vi "reconstruction_error.vi"(8 "error in (no error)":errorcluster caption="entrée d'erreur (pas d'erreur)", 11 "Isomap.lvclass":refnum<class "Isomap.lvclass">) -> (0 "error out":errorcluster caption="sortie d'erreur", 2 "reconstruction_error":dbl, 3 "Isomap.lvclass 2":refnum<class "Isomap.lvclass">)   [LabVIEW 2020, in "Isomap.lvclass"]
doc: "Compute the reconstruction error for the embedding.\n\n Returns\n -------\n reconstruction_error : float\n\n Notes\n -----\n The cost function of an isomap embedding is\n\n ``E = frobenius_norm[K(D) - K(D_fit)] / n_samples``\n\n Where D is the matrix of distances for the input data X,\n D_fit is the matrix of distances for the output embedding X_fit,\n and K is the isomap kernel:\n\n ``K(D) = -0.5 * (I - 1/n_samples) * D^2 * (I - 1/n_samples)``"
uses:
  Isomap.lvclass
  C:/Users/cipop/TDF Dropbox/2_Technologies de France/1 - Services et Etudes/PLAIY/2 - DEV/PLAIYLAB/code/Python/Python.lvclass
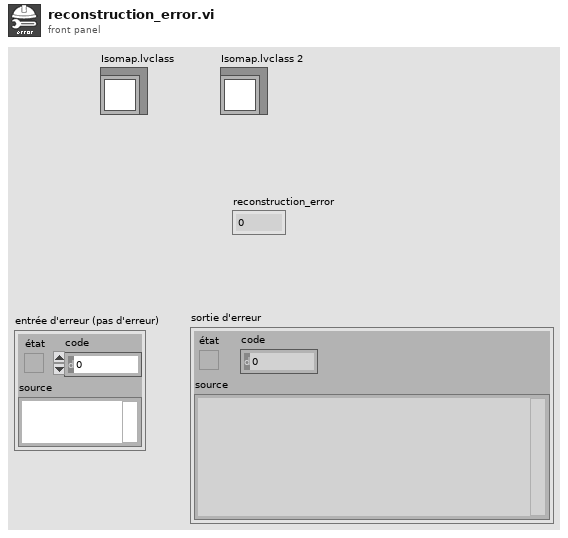
[diagram p1: front panel]
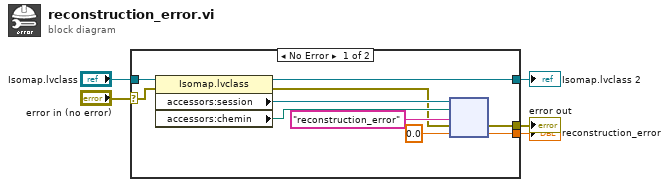
[diagram p0: block diagram]
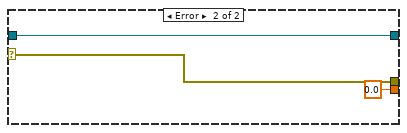
[diagram p2: hidden frame]
diagram:
  n1 = case shown="No Error" "error in (no error)" {
    selector: "error in (no error)" -> [w11 w18]
    tunnel: [w8 w18] -> w4
    tunnel: [w9 w17] -> w1
    tunnel: "Isomap.lvclass" -> [w14 w17]
    tunnel: [w6 0.0 ("Numeric")] -> w3
    frame No Error {
      n2 = property class="Isomap.lvclass"(reference=w14, error in=w11) -> (reference out=w9:refnum<class "Isomap.lvclass">, error out=w10:errorcluster, "accessors:session"=w13:refnum<k35>, "accessors:chemin"=w12:path)
      n3 = node(w13, w12, "reconstruction_error" ("nom de la fonction"), w10, 0.0 ("Numeric")) -> (w8:errorcluster, w6:dbl)  [unwired: 3 out]
    }
    frame Error {
    }
  }
  "error out" <- w4
  "reconstruction_error" <- w3
  "Isomap.lvclass 2" <- w1
